vi "Set_DAC.vi"(8 "Error in":errorcluster, 10 "appended array":u8[](array[numeric]), 11 "VISA Resource name":refnum<visa-resource-name>) -> (0 "error out":errorcluster, 3 "VISA resource name out":refnum<visa-resource-name>)   [LabVIEW 2015]
uses:
  MARS_Global_var.vi
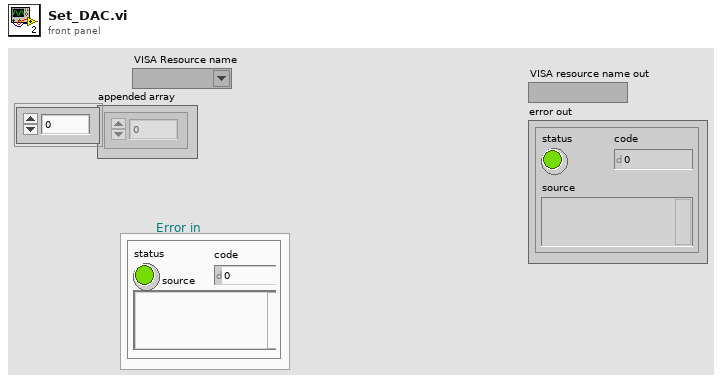
[diagram p1: front panel]
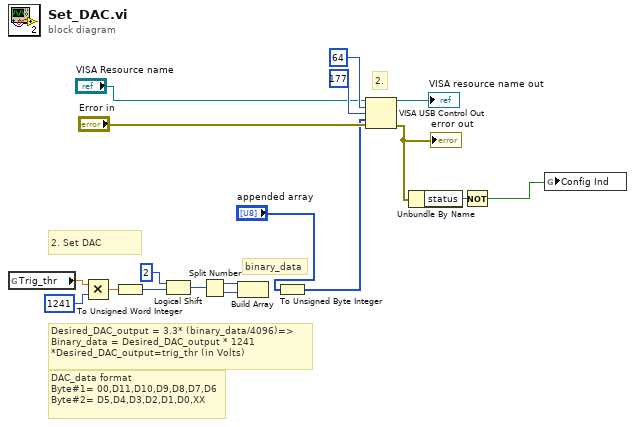
[diagram p0: block diagram]
diagram:
  # "2."
  # "binary_data"
  # "DAC_data format\nByte#1= 00,D11,D10,D9,D8,D7,D6\nByte#2= D5,D4,D3,D2,D1,D0,XX"
  # "Desired_DAC_output = 3.3* (binary_data/4096)=>\nBinary_data = Desired_DAC_output * 1241\n*Desired_DAC_output=trig_thr (in Volts)"
  # "2. Set DAC"
  n1 = global read "MARS_Global_var.vi" "Trig_thr"() -> (w10:dbl)
  n2 = Multiply(x=w10, y=1241) -> (x*y=w8:dbl)
  n3 = To Unsigned Word Integer(number=w8) -> (unsigned 16bit integer=w11:u16)
  n4 = Logical Shift(y=i16 2, x=w11) -> (x << y=w13:u16)
  n5 = Split Number(x=w13) -> (hi(x)=w14:u8, lo(x)=w15:u8)
  n6 = Build Array(w14, w15) -> ()  [unwired: 1 out]
  n7 = To Unsigned Byte Integer(number="appended array") -> (unsigned 8bit integer=w2:u8[])
  n8 = VISA USB Control Out(0:"VISA Resource name", 5:i16 64 ("request type"), 7:i16 177 ("request type"), 9:w2, 11:"Error in") -> (4:→"VISA resource name out":refnum<visa-resource-name>, 15:w7:errorcluster)  [unwired: 2 in]
  "error out" <- w7
  n9 = Unbundle By Name(w7) -> ("status"=w6:bool)
  n10 = Not(x=w6) -> (.not. x?=w3:bool)
  n11 = global write "MARS_Global_var.vi" "Config Ind"(w3) -> ()
